vi "create Pdf.vi"(6 "Bild-Qualität ( 0 = schlechteste, 1 = beste) 2":dbl(slide)=0.4954128440366973 min=0.0 max=1.0 scale=0.0..1.0, 7 "Data":T1={"Report.lvclass"=refnum, "Norm"="", "last State"=enum."Initialize", "Norm ID"=0, "parameter"=[], "EMTestCWS500N.lvclass"=refnum, "CEG4500.lvclass"=refnum, "Tektronix RSA5106A.lvclass"=refnum, "erfolgreich"=FALSE, "log"="", "Kommentar"="", "Device Enum"=enum."emTestCWS500N", "Test Enum"=enum."HF-Felder", "debug"=FALSE, "tab"=enum."Hauptmenü"}, 8 "Fehler (Eingang, kein Fehler)":errorcluster, 9 "wait until completion? (T)":bool=TRUE, 10 "Path":path=path "C:/Windows/System32", 11 "String (Eingang)":refnum<vi>) -> (0 "Fehler (Ausgang)":errorcluster, 1 "return code":i32 caption="Fehlercode", 2 "standard error":string caption="Standardfehler", 3 "standard output":string caption="Standardausgabe")   [LabVIEW 2013]
uses:
  Main/controls/Data.ctl
  classes/Datastructure/Report/Report.lvclass
  classes/Devices/emTestCWS500N/EMTestCWS500N.lvclass
  classes/Devices/CEG4500/CEG4500.lvclass
  classes/Devices/Tektronix RSA5106A/Tektronix RSA5106A.lvclass
  Main/controls/State.ctl
  classes/Devices/DeviceInterface/Devices.ctl
  classes/Tests/TestInterface/Tests.ctl
  Tabs.ctl
  lib/XML.lvlib
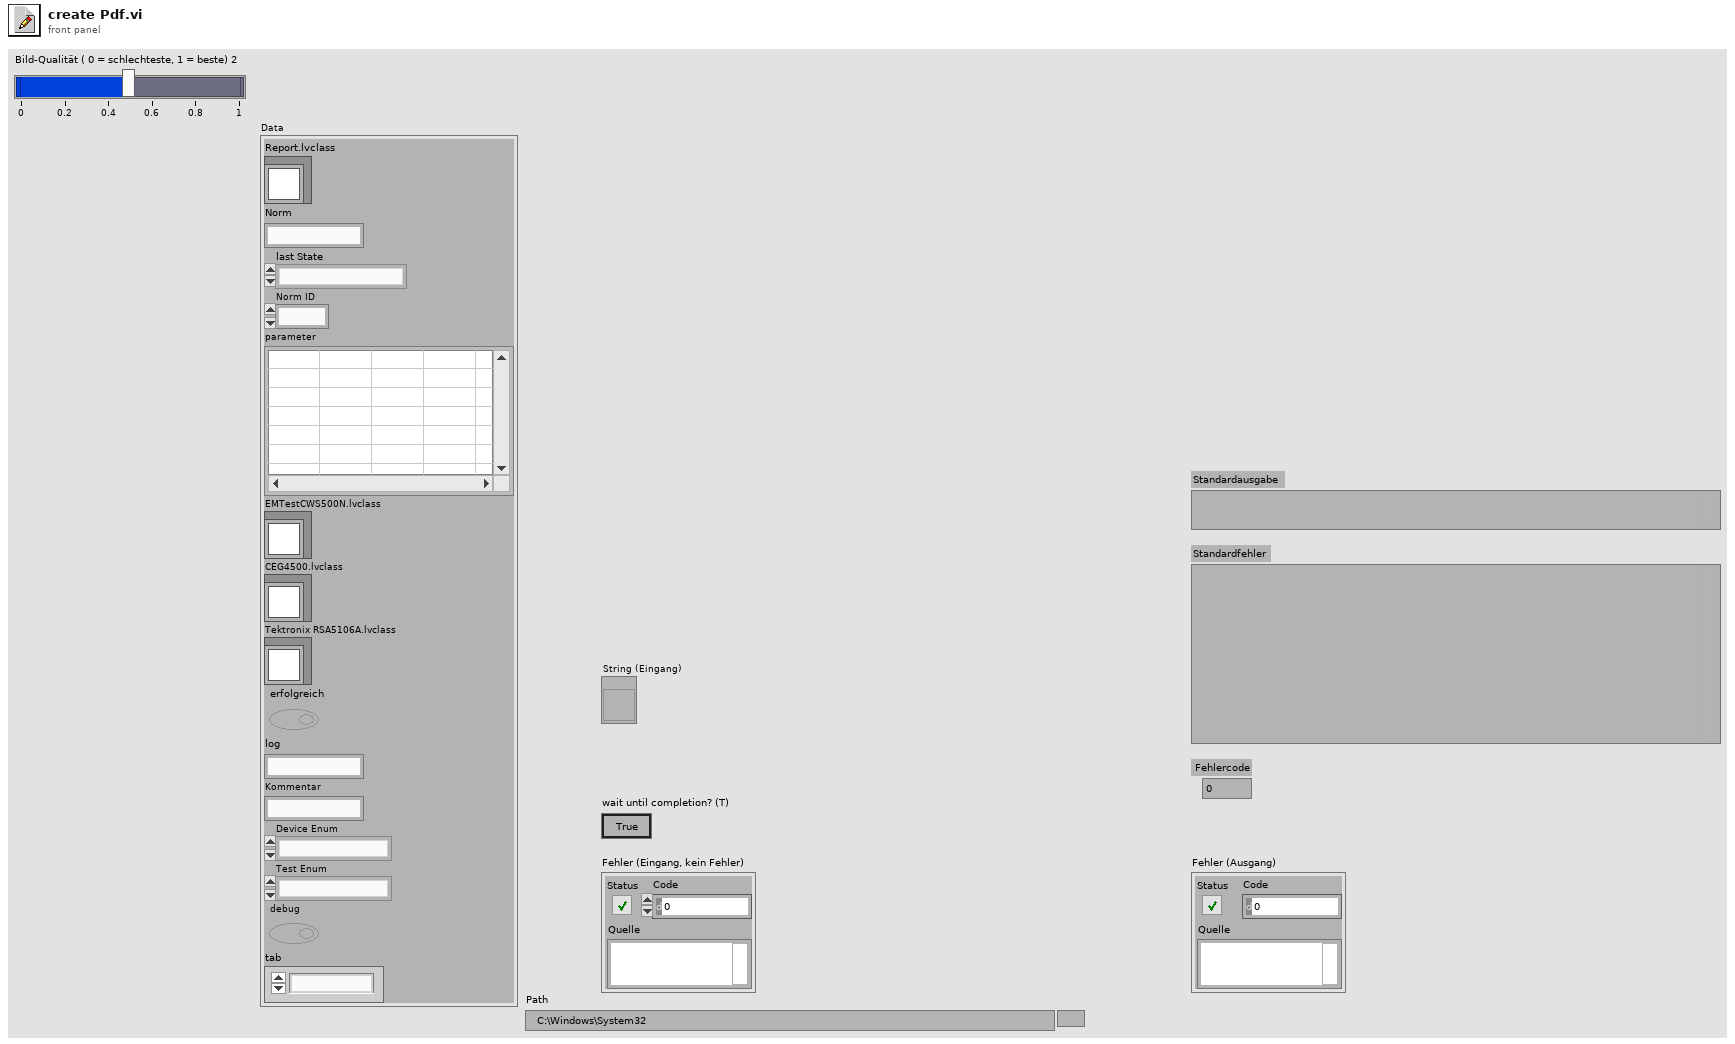
[diagram p1: front panel]
types:
  T1 = typedef "Data.ctl" = cluster{"Report.lvclass":refnum<class "Report.lvclass">, "Norm":string, "last State":T2, "Norm ID":i32, "parameter":string[][], "EMTestCWS500N.lvclass":refnum<class "EMTestCWS500N.lvclass">, "CEG4500.lvclass":refnum<class "CEG4500.lvclass">, "Tektronix RSA5106A.lvclass":refnum<class "Tektronix RSA5106A.lvclass">, "erfolgreich":bool, "log":string, "Kommentar":string, "Device Enum":T3, "Test Enum":T4, "debug":bool, "tab":T5}
  T2 = typedef "State.ctl" = enum16{"create Pdf", "load Report", "save Report", "do Test", "CDN Kalibrierung", "enter Report Parameters", "new Test", "Protokoll", "read Tree", "update Tree", "Fehler", "Initialize", "Wait for Event", "Exit"}
  T3 = typedef "Devices.ctl" = enum16{"unbekannt", "Tektronix RSA5106A", "emTestCWS500N", "CEG-4500"}
  T4 = typedef "Tests.ctl" = enum16{"unbekannt", "Störaussendung", "Burst", "ESD", "Surge", "Spannungseinbruch", "HF-Felder"}
  T5 = typedef "Tabs.ctl" = enum32{"Hauptmenü", "Prüfbericht", "Einstellungen"}
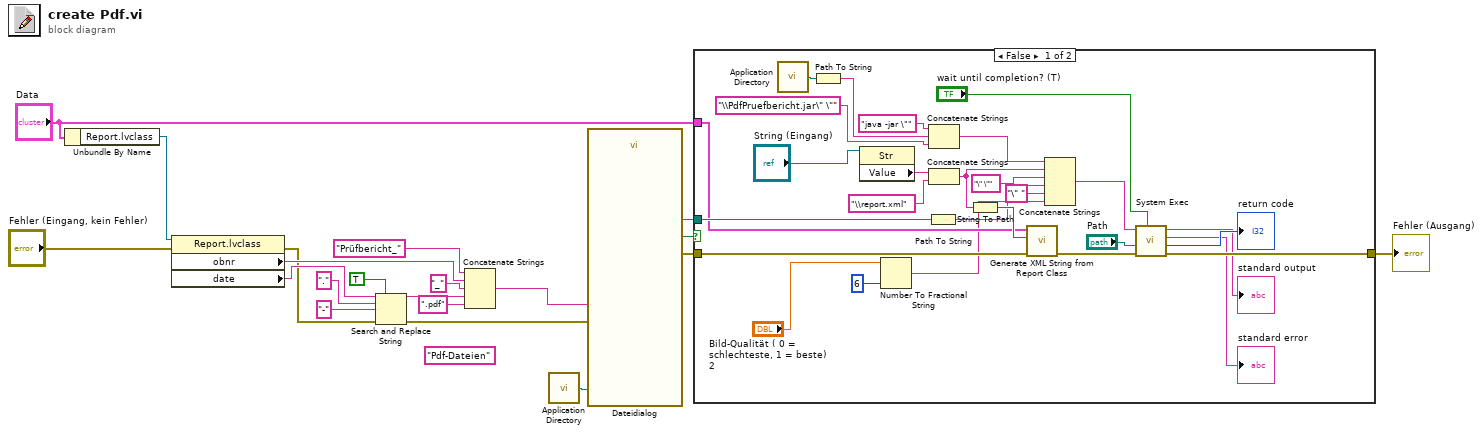
[diagram p0: block diagram]
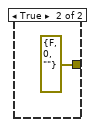
[diagram p2: hidden frame]
diagram:
  (unwired) "Pdf-Dateien" ("pattern label")
  n1 = Unbundle By Name("Data") -> ("Report.lvclass"=w15:refnum<class "Report.lvclass">)
  n2 = property class="Report.lvclass"(reference=w15, error in="Fehler (Eingang, kein Fehler)") -> (error out=w4:errorcluster, "obnr"=w13:string, "date"=w10:string)  [unwired: 1 out]
  n3 = Search and Replace String(replace all?=TRUE ("replace all? (F)"), input string=w10, search string=".", replace string="-" ("replace string (\"\")"), error in=w4) -> (result string=w7:string, error out=w6:errorcluster)  [unwired: 3 in, 2 out]
  n4 = Concatenate Strings("Prüfbericht_" ("string"), w13, "_" ("string"), w7, ".pdf" ("string")) -> (w11:string)
  n5 = call <vilib>:"Application Directory.vi"() -> ("Application Directory"=w2:path)
  n6 = call "Dateidialog"("start path"=w2, "default name"=w11, "error in"=w6) -> ("selected path"=w20:path, "cancelled"=w17:bool, "error out"=w19:errorcluster)  [unwired: 9 in, 1 out]
  n7 = case shown="False" w17 {
    tunnel: w20 -> [w41 _]
    tunnel: w19 -> [w40 _]
    tunnel: [w39 errorcluster {"status"=FALSE, "code"=0, "source"=""} ("error out")] -> w18
    tunnel: "Data" -> [w37 _]
    frame False {
      n8 = call <vilib>:"Application Directory.vi"() -> ("Application Directory"=w26:path)
      n9 = Path To String(path=w26) -> (string=w31:string)
      n10 = property class="Str"(reference="String (Eingang)") -> ("Value"=w42:string)  [unwired: 1 in, 2 out]
      n11 = Number To Fractional String(number="Bild-Qualität ( 0 = schlechteste, 1 = beste) 2", precision (6)=i16 6) -> (F-format string=w24:string)  [unwired: 2 in]
      n12 = Path To String(path=w41) -> (string=w44:string)
      n13 = Concatenate Strings("java -jar \"" ("command line"), w31, "\\PdfPruefbericht.jar\" \"") -> (w29:string)
      n14 = Concatenate Strings(w42, "\\report.xml") -> (w45:string)
      n15 = String To Path(string=w45) -> (path=w46:path)
      n16 = call "Generate XML String from Report Class.vi"("error in (no error)"=w40, "Dateipfad (Dialog verwenden)"=w46, "Daten"=w37) -> ("Fehler (Ausgang)"=w38:errorcluster)  [unwired: 8 in]
      n17 = Concatenate Strings(w29, w45, "\" \"" ("String"), w44, "\" " ("string"), w24) -> (w47:string)
      n18 = call <vilib>:"System Exec.vi"("wait until completion? (T)"="wait until completion? (T)", "error in (no error)"=w38, "working directory"="Path", "command line"=w47) -> ("error out"=w39:errorcluster, "return code"=→"return code":i32, "standard error"=→"standard error":string, "standard output"=→"standard output":string)  [unwired: 4 in]
    }
    frame True {
    }
  }
  "Fehler (Ausgang)" <- w18
